vi "all_in_one.vi"(4 "Frequency":i32=25000, 6 "Channel":i32=1, 7 "Duty Cycle":i32(knob) scale=0.0..100.0, 9 "reference":refnum<vi>, 10 "reference 2":refnum<vi>, 11 "Digital in":refnum<vi>) -> (0 "Numeric 4":dbl, 1 "Numeric":dbl, 2 "Numeric 2":dbl, 3 "Card Status":bool, 5 "Numeric 3":dbl)   [LabVIEW 2021]
uses:
  CHIDClass.dll
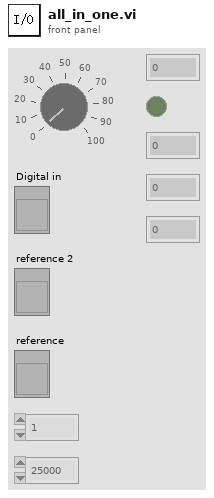
[diagram p1: front panel]
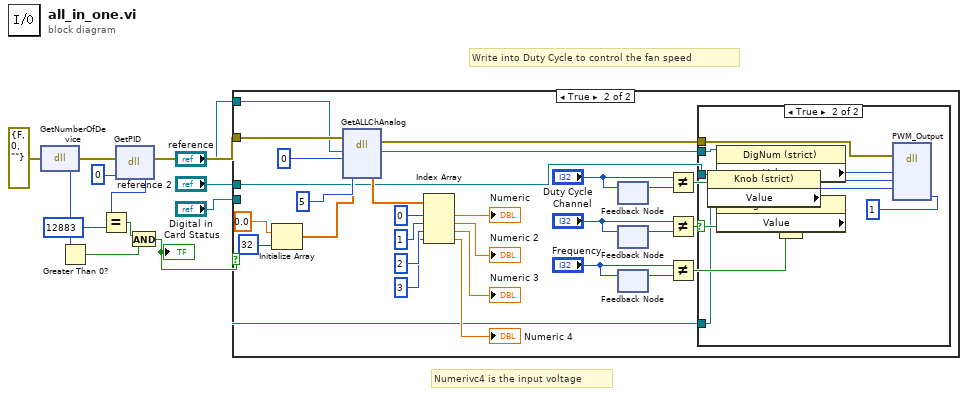
[diagram p0: block diagram]
diagram:
  # "Write into Duty Cycle to control the fan speed"
  # "Numerivc4 is the input voltage"
  n1 = dll-call lib="C:/Users/cheng/Desktop/CourseworkAI/CHIDClass.dll" fn="GetNumberOfDevice"(error in=errorcluster {"status"=FALSE, "code"=0, "source"=""} ("错误输入（无错误）")) -> (error out=w6:errorcluster, "result"=w7:i32)  [unwired: 2 in, 1 out]
  n2 = Greater Than 0?(x=w7) -> (x > 0?=w11:bool)
  n3 = dll-call lib="C:/Users/cheng/Desktop/CourseworkAI/CHIDClass.dll" fn="GetPID"(error in=w6, "i"=0) -> (error out=w13:errorcluster, "result"=w8:u16)  [unwired: 3 in, 1 out]
  n4 = Equal?(x=w8, y=12883 ("i")) -> (x = y?=w10:bool)
  n5 = And(x=w10, y=w11) -> (x .and. y?=w12:bool)
  "Card Status" <- w12
  n6 = case shown="True" w12 {
    tunnel: w13 -> [_ w42]
    tunnel: "reference" -> [_ w16]
    tunnel: "reference 2" -> [_ w15]
    tunnel: "Digital in" -> [_ w14]
    frame False {
    }
    frame True {
      n7 = Initialize Array(0.0 ("元素"), 32 ("维数大小")) -> (w37:dbl[])
      n8 = dll-call lib="C:/Users/cheng/Desktop/CourseworkAI/CHIDClass.dll" fn="GetALLChAnalog"(error in=w42, "mode"=0, "range"=5, "readBuffer"=w37) -> (error out=w17:errorcluster, "readBuffer"=w32:dbl[])  [unwired: 5 in, 1 out]
      n9 = Index Array(array=w32, index #1=0 ("索引"), index #2=1 ("索引"), index #3=2 ("索引"), index #4=3 ("索引")) -> (element #1=→"Numeric":dbl, element #2=→"Numeric 2":dbl, element #3=→"Numeric 3":dbl, element #4=→"Numeric 4":dbl)
      n10 = feedback #1() -> (w24:i32)  [unwired: 1 in]
      n11 = feedback-in #1("Duty Cycle") -> ()
      n12 = feedback #2() -> (w25:i32)  [unwired: 1 in]
      n13 = feedback-in #2("Channel") -> ()
      n14 = feedback #3() -> (w26:i32)  [unwired: 1 in]
      n15 = feedback-in #3("Frequency") -> ()
      n16 = Not Equal?(x="Duty Cycle", y=w24) -> (x != y?=w21:bool)
      n17 = Not Equal?(x="Channel", y=w25) -> (x != y?=w20:bool)
      n18 = Not Equal?(x="Frequency", y=w26) -> (x != y?=w19:bool)
      n19 = Compound Arithmetic op=OR(w21, w20, w19) -> (w18:bool)
      n20 = case shown="True" w18 {
        tunnel: w17 -> [_ w46]
        tunnel: w16 -> [_ w45]
        tunnel: w15 -> [_ w44]
        tunnel: w14 -> [_ w43]
        frame False {
        }
        frame True {
          n21 = property class="Knob (strict)"(reference=w44) -> ("Value"=w49:i32)  [unwired: 1 in, 2 out]
          n22 = property class="DigNum (strict)"(reference=w45) -> ("Value"=w50:i32)  [unwired: 1 in, 2 out]
          n23 = property class="DigNum (strict)"(reference=w43) -> ("Value"=w47:i32)  [unwired: 1 in, 2 out]
          n24 = dll-call lib="C:/Users/cheng/Desktop/CourseworkAI/CHIDClass.dll" fn="PWM_Output"(error in=w46, "fre"=w50, "dutyCyle"=w49, "ch"=w47, "isOpen"=1) -> ()  [unwired: 7 in, 2 out]
        }
      }
    }
  }
